vi "First.vi"(7 "Address":string, 8 "Error In":errorcluster) -> (0 "Error Out":errorcluster)   [LabVIEW 2017, in "Tests.lvlib" / "KnownHosts.lvlib"]
uses:
  KnownHosts.lvlib
  src/Toolkit/API/KnownHosts/API/Typedefs/Get Results.ctl
  <vilib>/Utility/error.llb/Clear Errors.vi
  <vilib>/Utility/file.llb/Is Path and Not Empty.vi
  <vilib>/Utility/sysdir.llb/Get System Directory.vi
  <vilib>/addons/_JKI Toolkits/Caraya/classes/Test/Test.lvclass
  <vilib>/addons/_JKI Toolkits/Caraya/classes/Assert/Assert.lvclass
  src/Toolkit/API/KnownHosts/KnownHosts.lvclass
  Tests.lvlib
  src/Toolkit/API/Session/Session.lvclass
  src/Toolkit/API/KnownHost/KnownHost.lvclass
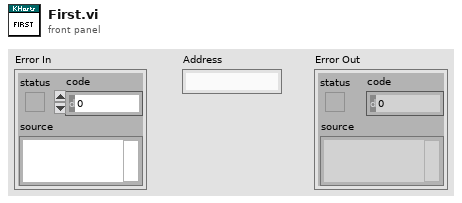
[diagram p1: front panel]
types:
  T1 = typedef "Toolkit.lvlib/KnownHosts.lvclass/Get Results.ctl" = enum32{"Success", "End of Hosts"}
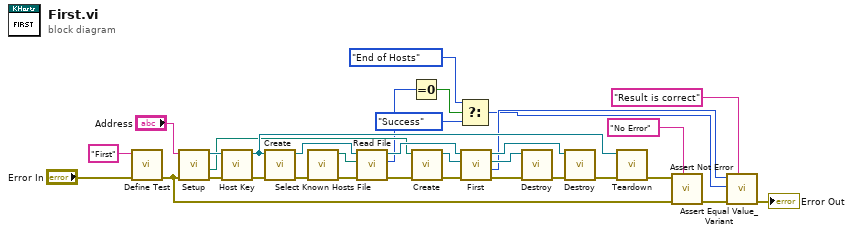
[diagram p0: block diagram]
diagram:
  n1 = call <vilib>:"Define Test.vi"("error in (no error)"="Error In", "Label (VI Title)"="First") -> ("error out"=w20:errorcluster)  [unwired: 9 in]
  n2 = call "Setup.vi"("Error In"=w20, "Address In"="Address") -> ("Error Out"=w21:errorcluster, "lv-libssh2 Shared Library"=w7:path, "Sesssion"=w22:refnum<class "Session.lvclass">)  [unwired: 6 in, 1 out]
  n3 = call "Host Key.vi"("Error In"=w21, "Session In"=w22) -> ("Error Out"=w23:errorcluster, "Sesssion Out"=w18:refnum<class "Session.lvclass">)  [unwired: 6 in, 2 out]
  n4 = call "Create.vi"("Error In"=w23, "Session"=w18) -> ("Error Out"=w29:errorcluster, "Known Hosts"=w30:refnum<class "KnownHosts.lvclass">)  [unwired: 8 in]
  n5 = call "Select Known Hosts File.vi"("Error In"=w29) -> ("Error Out"=w28:errorcluster, "Known Hosts File"=w27:path)  [unwired: 9 in]
  n6 = call "Read File.vi"("Error In"=w28, "File"=w27, "KnownHosts In"=w30) -> ("Error Out"=w12:errorcluster, "Count"=w5:u64, "KnownHosts Out"=w15:refnum<class "KnownHosts.lvclass">)  [unwired: 6 in]
  n7 = Equal To 0?(x=w5) -> (x = 0?=w4:bool)
  n8 = call "Create.vi"("Error In"=w12, "lv-libssh2 Shared Library"=w7) -> ("Error Out"=w11:errorcluster, "Known Host"=w13:refnum<class "KnownHost.lvclass">)  [unwired: 8 in]
  n9 = Select(t=Get_Results."End of Hosts" ("Get Result"), s=w4, f=Get_Results."Success" ("Get Result")) -> (s? t:f=w1:T1)
  n10 = call "First.vi"("Error In"=w11, "Known Host In"=w13, "KnownHosts In"=w15) -> ("Error Out"=w9:errorcluster, "Result"=w6:T1, "Known Host Out"=w10:refnum<class "KnownHost.lvclass">, "KnownHosts Out"=w14:refnum<class "KnownHosts.lvclass">)  [unwired: 5 in]
  n11 = call "Destroy.vi"("Error In"=w9, "Known Host"=w10) -> ("Error Out"=w8:errorcluster)  [unwired: 8 in, 1 out]
  n12 = call "Destroy.vi"("Error In"=w8, "KnownHosts"=w14) -> ("Error Out"=w17:errorcluster)  [unwired: 8 in, 1 out]
  n13 = call "Teardown.vi"("Error In"=w17, "Session"=w18) -> ("Error Out"=w16:errorcluster)  [unwired: 9 in]
  n14 = call <vilib>:"Assert Not Error.vi"("Label"="No Error", "error in (no error)"=w20, "Not Error?"=w16) -> ("error out"=w26:errorcluster)  [unwired: 8 in]
  n15 = call <vilib>:"Assert Equal Value_Variant.vi"("Label"="Result is correct", "error in (no error)"=w26, "Y"=w1, "X"=w6) -> ("error out"=→"Error Out":errorcluster)  [unwired: 7 in]
